vi "EditLine.vi"() -> ()   [LabVIEW 2020, in "Curve Editor.lvlib"]
uses:
  Curve Editor.lvlib
  Key Value/Key Value.lvlib
panel:
  in  "终点值":dbl format="%.2f"
  in  "起点值":dbl format="%.2f"
  in  "时间[S]":dbl format="%.2f"
  in  "Tree引用句柄":refnum<vi>
  in  "索引":i32
  in  "取消按钮":bool
  in  "确定按钮":bool
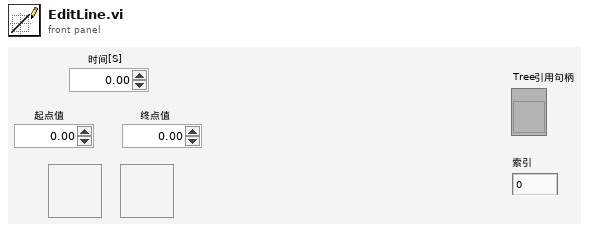
[diagram p1: front panel]
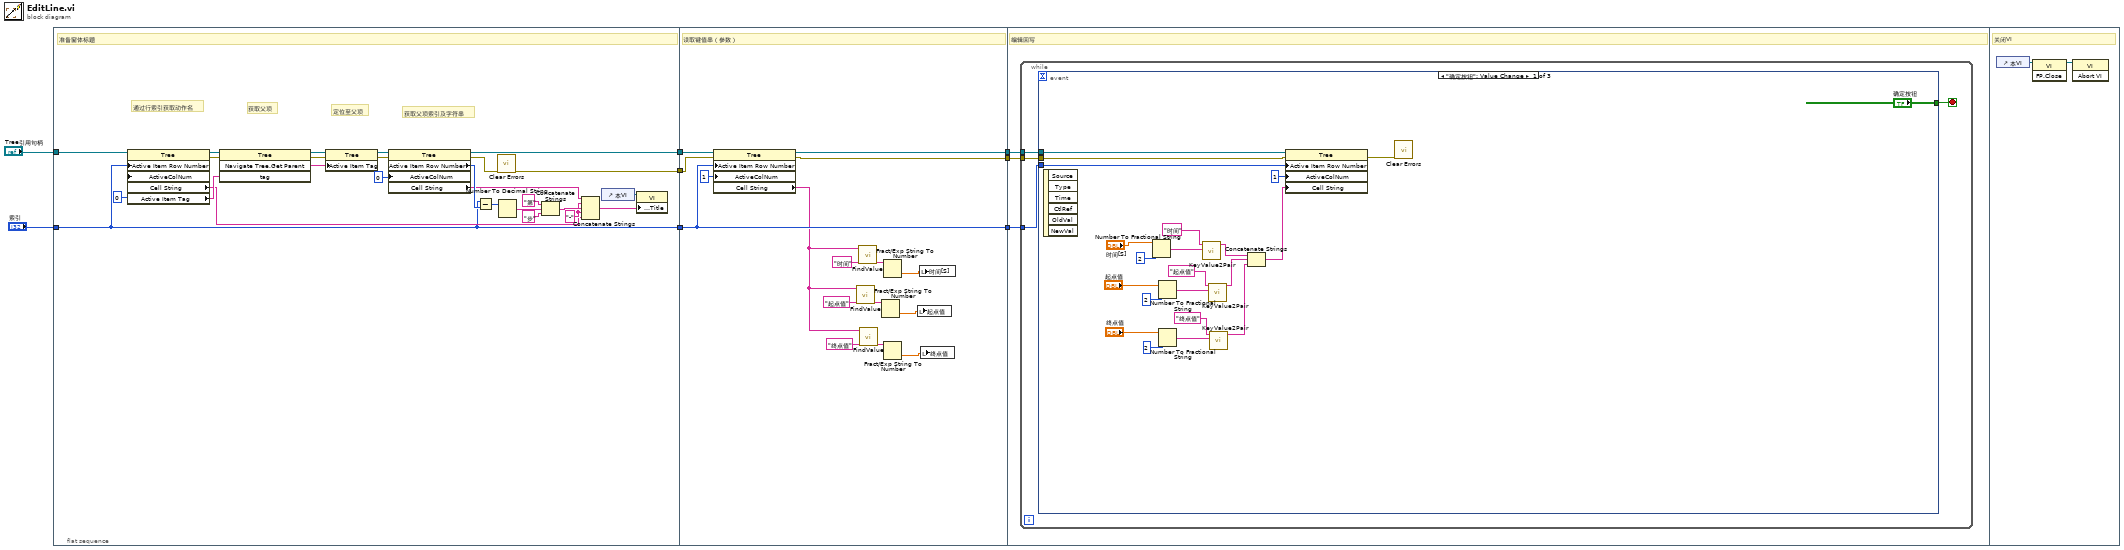
[diagram p0: block diagram]
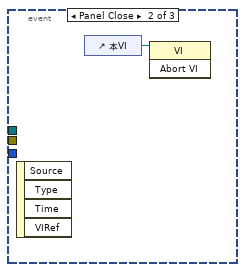
[diagram p2: hidden frame]
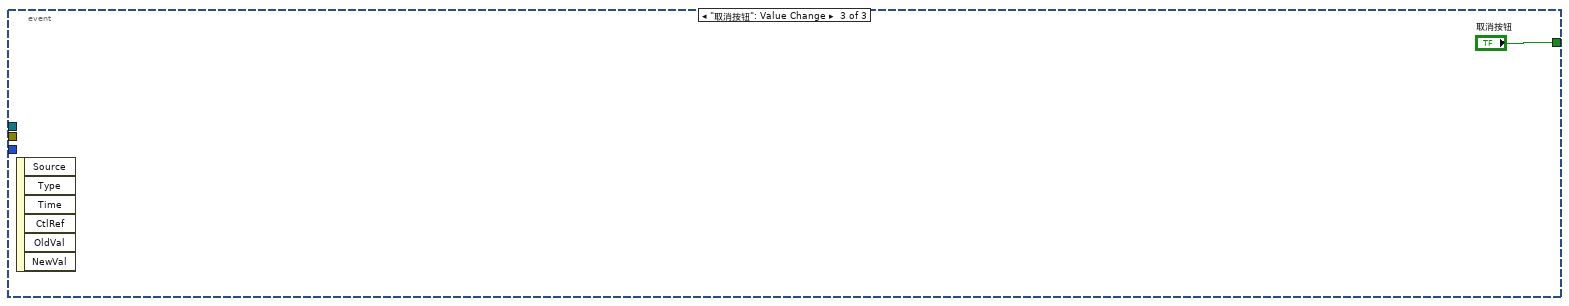
[diagram p3: hidden frame]
diagram:
  n1 = flat-sequence {
    tunnel: [w16] -> w8
    tunnel: [w15] -> w6
    tunnel: "Tree引用句柄" -> [w17]
    tunnel: "索引" -> [w16]
    tunnel: [w9] -> w2
    tunnel: w8 -> [w48]
    tunnel: [w48] -> w7
    tunnel: w6 -> [w49]
    tunnel: [w47] -> w5
    tunnel: w2 -> [w36]
    tunnel: [w35] -> w1
    tunnel: w7 -> [w53]
    tunnel: w5 -> [w52]
    tunnel: w1 -> [w51]
    frame #0 {
      w19 = "-" ("字符串")
      # "获取父项索引及字符串"
      # "定位至父项"
      # "获取父项"
      # "通过行索引获取动作名"
      # "准备窗体标题"
      n2 = property class="Tree"(reference=w17, "Active Item Row Number"=w16, "ActiveColNum"=0 ("活动单元格:活动列数")) -> (reference out=w14:refnum<vi>, error out=w13:errorcluster, "Cell String"=w18:string, "Active Item Tag"=w31:string)  [unwired: 1 in]
      n3 = invoke class="Tree" method="Navigate Tree.Get Parent"(reference=w14, error in=w13, "tag"=w31) -> (reference out=w26:refnum<vi>, error out=w12:errorcluster, "Navigate Tree:Get Parent"=w27:string)  [unwired: 1 in, 1 out]
      n4 = property class="Tree"(reference=w26, error in=w12, "Active Item Tag"=w27) -> (reference out=w25:refnum<vi>, error out=w11:errorcluster)
      n5 = property class="Tree"(reference=w25, error in=w11, "ActiveColNum"=0 ("活动单元格:活动列数")) -> (reference out=w15:refnum<vi>, error out=w10:errorcluster, "Active Item Row Number"=w29:i32, "Cell String"=w28:string)
      n6 = Subtract(x=w16, y=w29) -> (x-y=w24:i32)
      n7 = call <vilib>:"Clear Errors.vi"("error in (no error)"=w10) -> ("error out"=w9:errorcluster)  [unwired: 5 in, 1 out]
      n8 = Number To Decimal String(number=w24) -> (decimal integer string=w22:string)  [unwired: 1 in]
      n9 = Concatenate Strings("第", w22, "步") -> (w20:string)
      n10 = Concatenate Strings(w28, w19, w20, w19, w18) -> (w32:string)
      n11 = control-ref of="本VI"() -> (w34:refnum<vi>)
      n12 = property class="VI"(reference=w34, "Front Panel.Title"=w32) -> ()  [unwired: 1 in, 2 out]
    }
    frame #1 {
      # "读取键值串（参数）"
      n13 = property class="Tree"(reference=w49, error in=w36, "Active Item Row Number"=w48, "ActiveColNum"=1 ("活动单元格:活动列数")) -> (reference out=w47:refnum<vi>, error out=w35:errorcluster, "Cell String"=w37:string)
      n14 = call "FindValue.vi"("键"="起点值", "键值串"=w37) -> ("值"=w42:string)  [unwired: 8 in, 1 out]
      n15 = call "FindValue.vi"("键"="时间", "键值串"=w37) -> ("值"=w45:string)  [unwired: 8 in, 1 out]
      n16 = call "FindValue.vi"("键"="终点值", "键值串"=w37) -> ("值"=w39:string)  [unwired: 8 in, 1 out]
      n17 = Fract/Exp String To Number(string=w42) -> (number=w43:dbl)  [unwired: 3 in, 1 out]
      n18 = Fract/Exp String To Number(string=w45) -> (number=w44:dbl)  [unwired: 3 in, 1 out]
      n19 = Fract/Exp String To Number(string=w39) -> (number=w38:dbl)  [unwired: 3 in, 1 out]
      n20 = local write "起点值"(w43) -> ()
      n21 = local write "时间[S]"(w44) -> ()
      n22 = local write "终点值"(w38) -> ()
    }
    frame #2 {
      # "编辑回写"
      n23 = while {
        tunnel: w53 -> [w56]
        tunnel: w52 -> [w55]
        tunnel: w51 -> [w54]
        stop <- w57 stop-if-true
        n24 = event shown="[0] \"确定按钮\": Value Change" {
          selector: _ -> [_ _ _]
          dyn-events: _ -> [_ _ _]
          timeout: _ -> [_ _ _]
          tunnel: ["确定按钮" _ "取消按钮"] -> w57
          tunnel: w56 -> [w78 _ _]
          tunnel: w55 -> [w77 _ _]
          tunnel: w54 -> [w59 _ _]
          event "确定按钮": Value Change {
            n25 = event-data() -> ()  [unwired: 1 in, 6 out]
            n26 = Number To Fractional String(number="时间[S]", precision (6)=i16 2 ("精度(6)")) -> (F-format string=w74:string)  [unwired: 2 in]
            n27 = Number To Fractional String(number="起点值", precision (6)=i16 2 ("精度(6)")) -> (F-format string=w71:string)  [unwired: 2 in]
            n28 = Number To Fractional String(number="终点值", precision (6)=i16 2 ("精度(6)")) -> (F-format string=w68:string)  [unwired: 2 in]
            n29 = call "KeyValue2Pair.vi"("值"=w74, "键"="时间") -> ("键值对"=w63:string)  [unwired: 9 in]
            n30 = call "KeyValue2Pair.vi"("值"=w71, "键"="起点值") -> ("键值对"=w62:string)  [unwired: 9 in]
            n31 = call "KeyValue2Pair.vi"("值"=w68, "键"="终点值") -> ("键值对"=w61:string)  [unwired: 9 in]
            n32 = Concatenate Strings(w63, w62, w61) -> (w60:string)
            n33 = property class="Tree"(reference=w77, error in=w59, "Active Item Row Number"=w78, "ActiveColNum"=1 ("活动单元格:活动列数"), "Cell String"=w60) -> (error out=w58:errorcluster)  [unwired: 1 out]
            n34 = call <vilib>:"Clear Errors.vi"("error in (no error)"=w58) -> ()  [unwired: 5 in, 2 out]
          }
          event Panel Close {
            n35 = event-data() -> ()  [unwired: 1 in, 4 out]
            n36 = control-ref of="本VI"() -> (w80:refnum<vi>)
            n37 = invoke class="VI" method="Abort VI"(reference=w80) -> ()  [unwired: 2 in, 3 out]
          }
          event "取消按钮": Value Change {
            n38 = event-data() -> ()  [unwired: 1 in, 6 out]
          }
        }
      }
    }
    frame #3 {
      # "关闭VI"
      n39 = control-ref of="本VI"() -> (w83:refnum<vi>)
      n40 = invoke class="VI" method="FP.Close"(reference=w83) -> (reference out=w82:refnum<vi>)  [unwired: 2 in, 2 out]
      n41 = invoke class="VI" method="Abort VI"(reference=w82) -> ()  [unwired: 2 in, 3 out]
    }
  }
